vi "PSVCH_Engine.vi"() -> ()   [LabVIEW 2016]
uses:
  Ctrls/PSVCH_VCH Info.ctl
  Ctrls/PSVCH_Status.ctl
  ToolKit/Formula/Ctrls/PSFormula_FOR_Formula Node.ctl
  ToolKit/Formula/Ctrls/PSFormula_FOR_Formula Step.ctl
  ToolKit/Formula/Ctrls/PSFormula_FOR_Formula Para.ctl
  ToolKit/Formula/Ctrls/PSFormula_FOR_Formula MidVar Data.ctl
  Ctrls/PSVCH_VarList.ctl
  Ctrls/PSVCH_Formula Node.ctl
  Ctrls/PSVCH_Formula Step.ctl
  Ctrls/PSVCH_Formula Para.ctl
  Ctrls/PSVCH_Formula MidVar Data.ctl
  Ctrls/PSVCH_VCH Status.ctl
  Architecture/Queue Management/ARC_Queue Create_Single.vi
  Architecture/Queue Management/ARC_Queue Valid.vi
  Architecture/Queue Management/ARC_Queue Remove Element.vi
  Architecture/Queue Management/ARC_Queue Insert Element.vi
  Architecture/Queue Management/ARC_Queue Destroy_Single.vi
panel:
  in  "Formula Node":T1
  in  "Q-Caller":string
  in  "TempVariable":T12
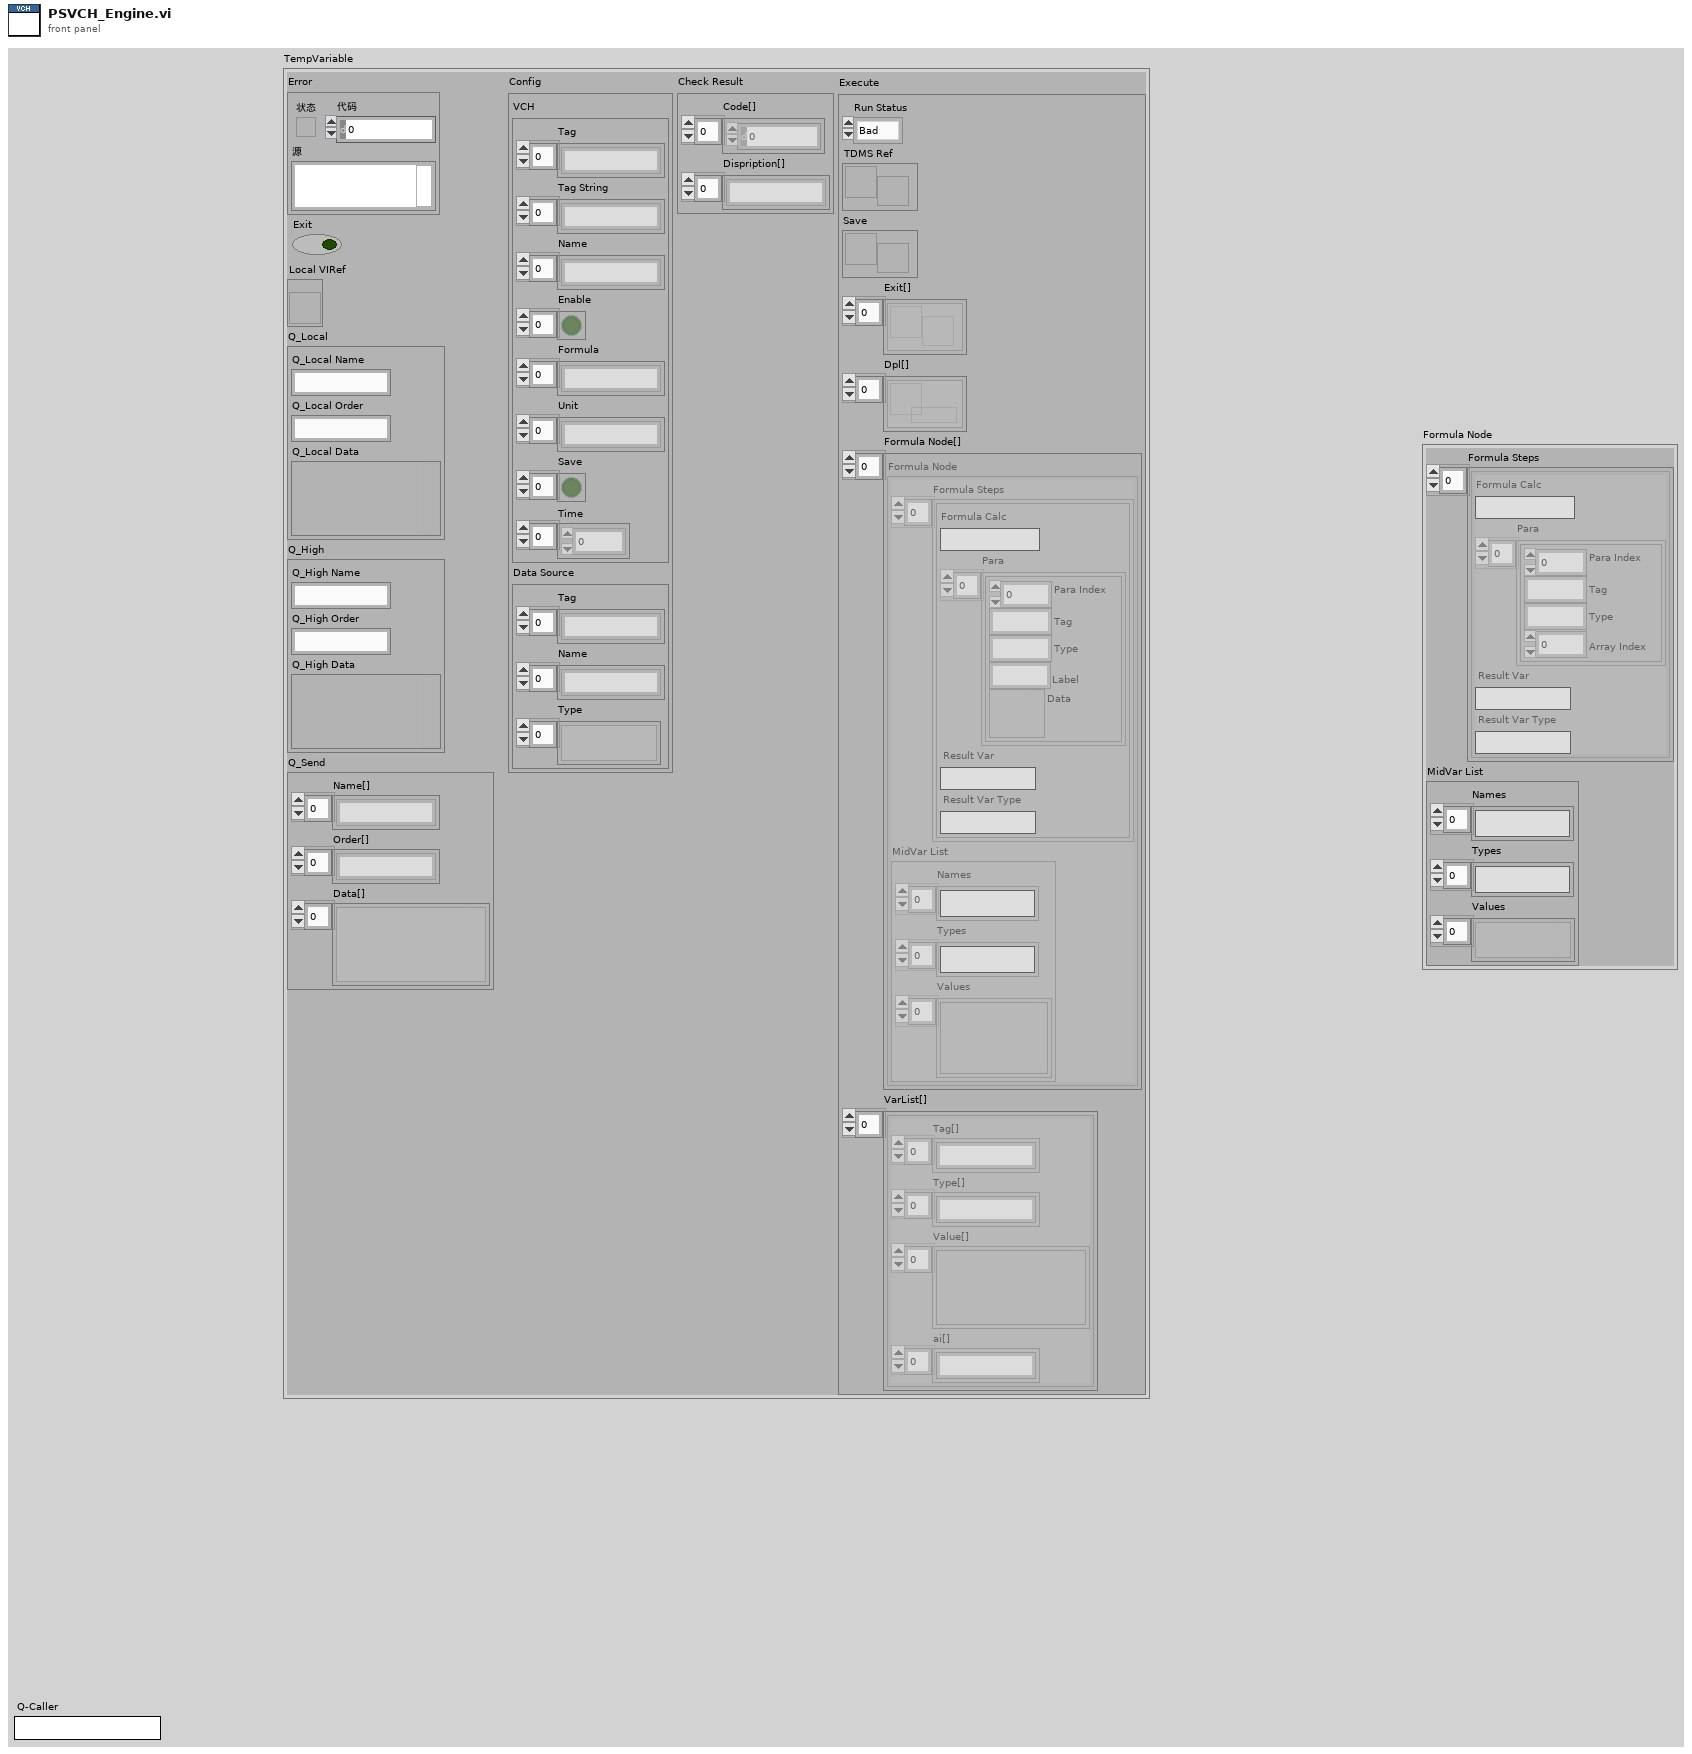
[diagram p1: front panel]
types:
  T1 = typedef "PSVCH_Formula Node.ctl" = cluster{"Formula Steps":T2[], "MidVar List":T4}
  T2 = typedef "PSVCH_Formula Step.ctl" = cluster{"Formula Calc":string, "Para":T3[], "Result Var":string, "Result Var Type":string}
  T3 = typedef "PSVCH_Formula Para.ctl" = cluster{"Para Index":i32, "Tag":string, "Type":string, "Array Index":i32}
  T4 = typedef "PSVCH_Formula MidVar Data.ctl" = cluster{"Names":string[], "Types":string[], "Values":variant[]}
  T5 = typedef "PSVCH_VCH Info.ctl" = cluster{"Tag":string[], "Tag String":string[], "Name":string[], "Enable":bool[], "Formula":string[], "Unit":string[], "Save":bool[], "Time":i64[]}
  T6 = typedef "PSVCH_Status.ctl" = enum16{"Bad", "Stop", "Run", "Pause"}
  T7 = typedef "PSFormula_FOR_Formula Node.ctl" = cluster{"Formula Steps":T8[], "MidVar List":T10}
  T8 = typedef "PSFormula_FOR_Formula Step.ctl" = cluster{"Formula Calc":string, "Para":T9[], "Result Var":string, "Result Var Type":string}
  T9 = typedef "PSFormula_FOR_Formula Para.ctl" = cluster{"Para Index":i32, "Tag":string, "Type":string, "Label":string, "Data":variant}
  T10 = typedef "PSFormula_FOR_Formula MidVar Data.ctl" = cluster{"Names":string[], "Types":string[], "Values":variant[]}
  T11 = typedef "PSVCH_VarList.ctl" = cluster{"Tag[]":string[], "Type[]":string[], "Value[]":variant[], "ai[]":string[]}
  T12 = cluster{"Error":errorcluster, "Exit":bool, "Local VIRef":refnum<vi>, "Q_Local":cluster{"Q_Local Name":string, "Q_Local Order":string, "Q_Local Data":variant}, "Q_High":cluster{"Q_High Name":string, "Q_High Order":string, "Q_High Data":variant}, "Q_Send":cluster{"Name[]":string[], "Order[]":string[], "Data[]":variant[]}, "Config":cluster{"VCH":T5, "Data Source":cluster{"Tag":string[], "Name":string[], "Type":variant[]}}, "Check Result":cluster{"Code[]":i32[], "Dispription[]":string[]}, "Execute":cluster{"Run Status":T6, "TDMS Ref":refnum<notifier>, "Save":refnum<notifier>, "Exit[]":refnum<notifier>[], "Dpl[]":refnum<queue>[], "Formula Node[]":T7[], "VarList[]":T11[]}}
  T13 = typedef "PSVCH_VCH Status.ctl" = cluster{"Tag":string[], "Code[]":i32[], "Dispription[]":string[]}
  T14 = cluster{"Q_High Name":string, "Tag":string, "t0":timestamp, "Period":i64, "Exit":refnum<notifier>, "Dpl":refnum<queue>, "TDMS Ref":refnum<notifier>, "Save":refnum<notifier>, "Formula Node 2":T7, "VarList":T11, "Save?":bool, "Name":string, "Unit":string}
  T15 = cluster{"Tag":string[], "Name":string[], "Type":variant[]}
  T16 = cluster{"Data Source":cluster{"Tag":string[], "Name":string[], "Type":variant[]}, "VCH":T5}
  T17 = cluster{"Q_Local Name":string, "Error":errorcluster}
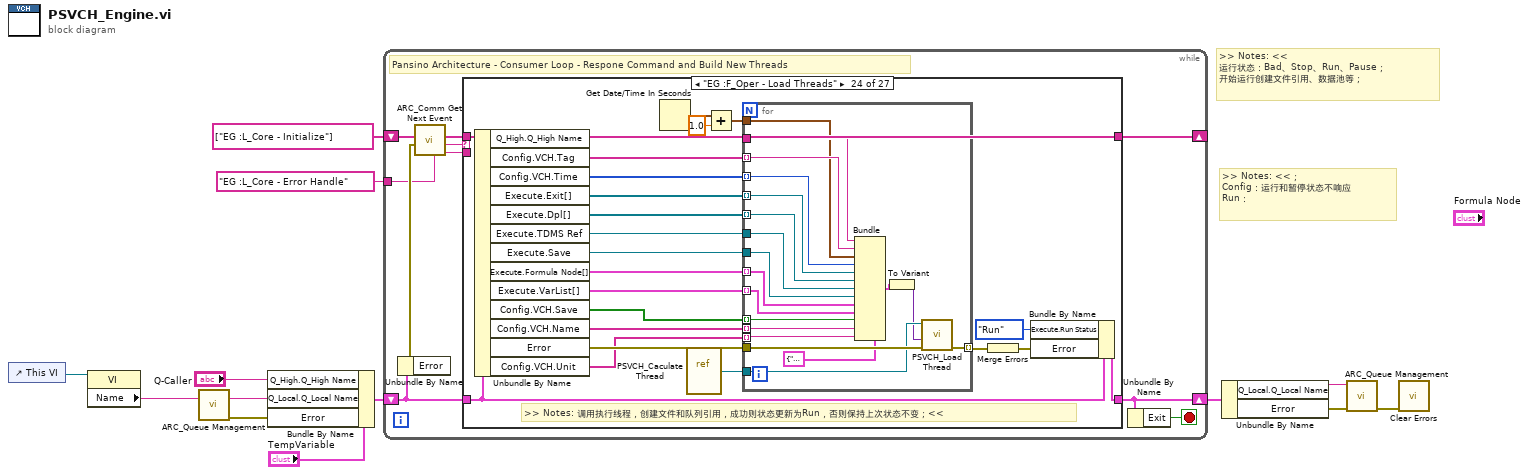
[diagram p0: block diagram]
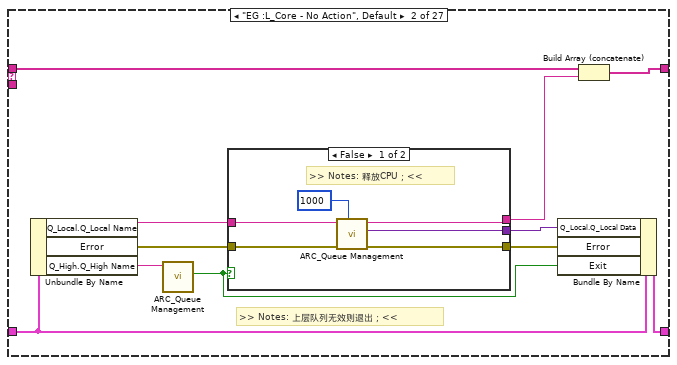
[diagram p3: hidden frame]
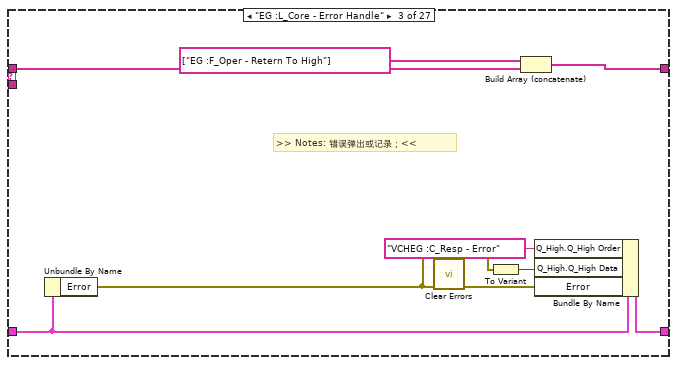
[diagram p5: hidden frame]
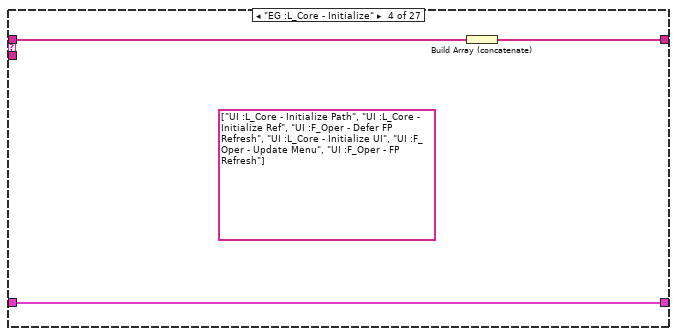
[diagram p6: hidden frame]
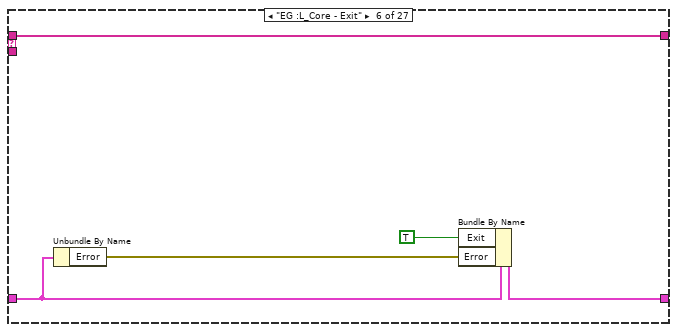
[diagram p8: hidden frame]
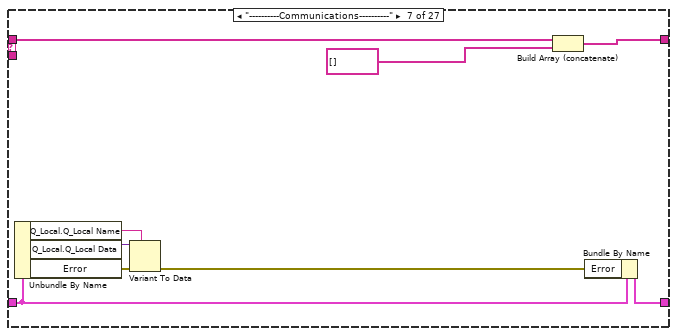
[diagram p9: hidden frame]
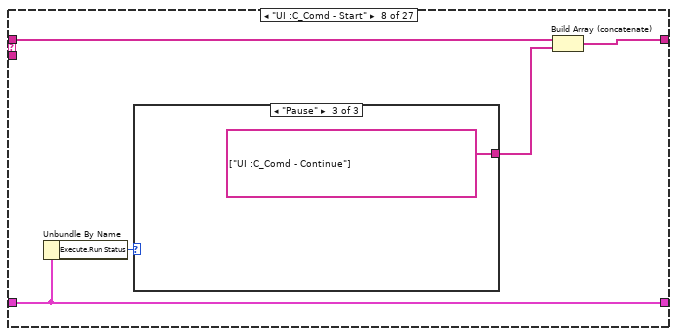
[diagram p10: hidden frame]
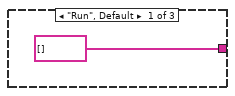
[diagram p11: hidden frame]
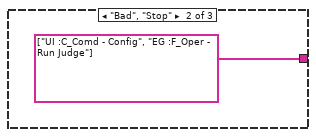
[diagram p12: hidden frame]
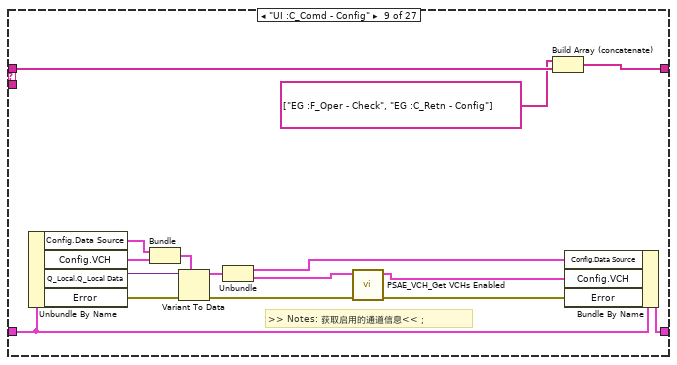
[diagram p13: hidden frame]
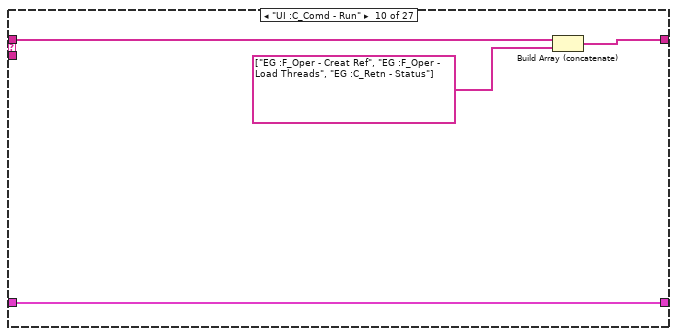
[diagram p14: hidden frame]
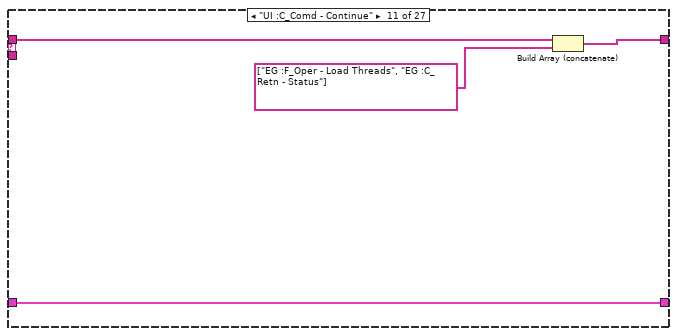
[diagram p15: hidden frame]
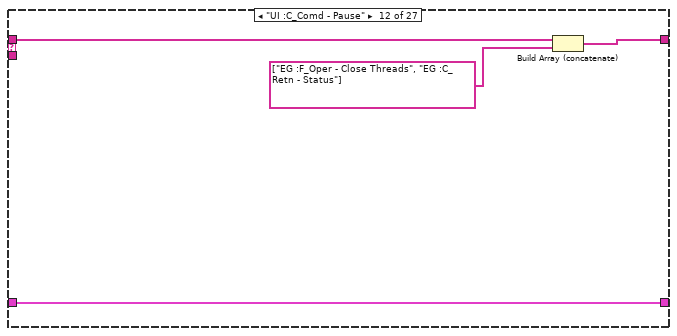
[diagram p16: hidden frame]
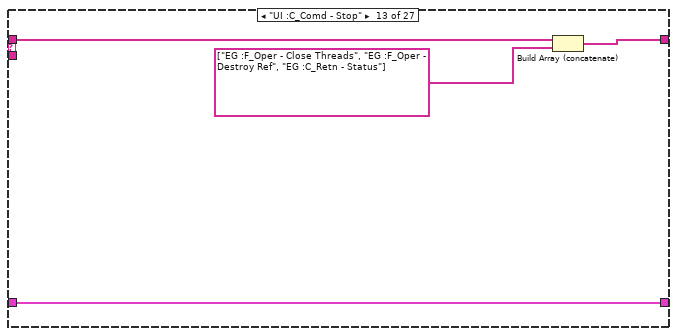
[diagram p17: hidden frame]
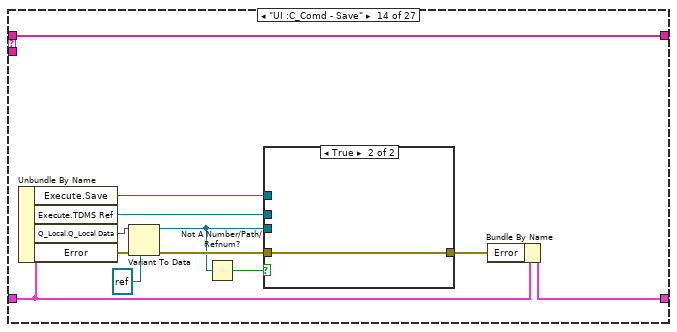
[diagram p18: hidden frame]
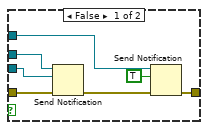
[diagram p19: hidden frame]
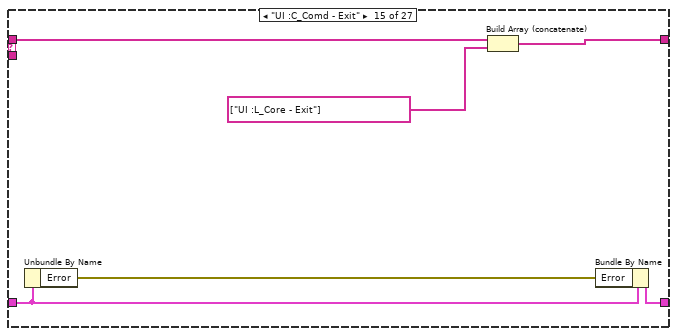
[diagram p20: hidden frame]
diagram:
  # ">> Notes: <<；\nConfig：运行和暂停状态不响应\nRun："
  # ">> Notes: <<\n运行状态：Bad、Stop、Run、Pause；\n开始运行创建文件引用、数据池等；"
  n1 = control-ref of="This VI"() -> (w2:refnum<vi>)
  n2 = property class="VI"(reference=w2) -> ("Name"=w1:string)  [unwired: 1 in, 2 out]
  n3 = call-poly "ARC_Queue Management.vi"("Queue Name"=w1) -> ("error out"=w3:errorcluster)  [unwired: 8 in, 2 out]
  n4 = Bundle By Name(cluster="TempVariable", "Q_High.Q_High Name"="Q-Caller", "Q_Local.Q_Local Name"=w1, "Error"=w3) -> (w11:T12)
  n5 = while {
    shift-right: [w16] -> w7
    shift-left: w11 -> [w18]
    shift-right: [w19] -> _
    shift-left: string[] ["EG :L_Core - Initialize"] -> [w22]
    tunnel: "EG :L_Core - Error Handle" ("Error Handle") -> [w14]
    stop <- w15 stop-if-true
    # "Pansino Architecture - Consumer Loop - Respone Command and Build New Threads"
    n6 = Unbundle By Name(w18) -> ("Error"=w17:errorcluster)
    n7 = call "ARC_Comm Get Next Event.vi"("Error Handle"=w14, "error in (no error)"=w17, "event queue in"=w22) -> ("prev event"=w13:string, "next event"=w21:string, "event queue out"=w20:string[])  [unwired: 3 in]
    n8 = case shown="\"EG :F_Oper - Load Threads\"" w21 {
      tunnel: w18 -> [w23 w32 w49 w53 w55 w58 w67 w72 w92 w95 w99 w103 w107 w121 w135 w148 w157 w171 w174 w183 w191 w225 w249 w279 w307 w327 w342]
      tunnel: w20 -> [w24 w30 w51 w54 w56 w61 w70 w75 w94 w98 w102 w106 w110 w122 w133 w149 w151 w160 w175 w184 w199 w223 w250 w282 w309 w328 w343]
      tunnel: [w24 w29 w45 w52 w56 w61 w69 w74 w93 w97 w101 w105 w109 w122 w132 w143 w150 w159 w175 w184 w199 w223 w250 w282 w309 w328 w337] -> w19
      tunnel: [w23 w31 w50 w53 w55 w59 w66 w72 w91 w95 w99 w103 w107 w119 w134 w147 w156 w170 w173 w182 w192 w224 w245 w280 w308 w323 w342] -> w16
      tunnel: w13 -> [_ _ _ _ _ _ _ _ _ _ _ _ _ _ _ _ _ _ _ _ _ _ _ _ _ _ _]
      frame "----------Core Status----------" {
      }
      frame "EG :L_Core - No Action", Default {
        # ">> Notes: 上层队列无效则退出；<<"
        n9 = Unbundle By Name(w32) -> ("Q_Local.Q_Local Name"=w27:string, "Error"=w33:errorcluster, "Q_High.Q_High Name"=w26:string)
        n10 = call-poly "ARC_Queue Management.vi"("Queue Name(unamed)"=w26) -> ("Not Exist?"=w25:bool)  [unwired: 8 in, 2 out]
        n11 = case shown="False" w25 {
          tunnel: [w41 w42] -> w35
          tunnel: [w40 _] -> w34
          tunnel: w33 -> [w39 w42]
          tunnel: [w38 _] -> w28
          tunnel: w27 -> [w37 _]
          frame False {
            # ">> Notes: 释放CPU；<<"
            n12 = call-poly "ARC_Queue Management.vi"("Time out(-1)_queue out"=1000, "error in (no error)"=w39, "Queue Name(unamed)"=w37) -> ("error out"=w41:errorcluster, "Data"=w40:variant, "Event"=w38:string)  [unwired: 5 in, 1 out]
          }
          frame True {
          }
        }
        n13 = Bundle By Name(cluster=w32, "Q_Local.Q_Local Data"=w34, "Error"=w35, "Exit"=w25) -> (w31:T12)
        n14 = Build Array (concatenate)(w30, w28) -> (w29:string[])
      }
      frame "EG :L_Core - Error Handle" {
        # ">> Notes: 错误弹出或记录；<<"
        n15 = Unbundle By Name(w49) -> ("Error"=w46:errorcluster)
        n16 = call <vilib>:"Clear Errors.vi"("error in (no error)"=w46) -> ("error out"=w47:errorcluster)  [unwired: 5 in, 1 out]
        n17 = To Variant(anything=w46) -> (Variant=w48:variant)
        n18 = Build Array (concatenate)(string[] ["EG :F_Oper - Retern To High"] ("数组"), w51) -> (w45:string[])
        n19 = Bundle By Name(cluster=w49, "Q_High.Q_High Order"="VCHEG :C_Resp - Error", "Q_High.Q_High Data"=w48, "Error"=w47) -> (w50:T12)
      }
      frame "EG :L_Core - Initialize" {
        (unwired) string[] ["UI :L_Core - Initialize Path", "UI :L_Core - Initialize Ref", "UI :F_Oper - Defer FP Refresh", "UI :L_Core - Initialize UI", "UI :F_Oper - Update Menu", "UI :F_Oper - FP Refresh"] ("数组")
        n20 = Build Array (concatenate)(w54) -> (w52:string[])
      }
      frame "EG :L_Core - Initialize Path" {
      }
      frame "EG :L_Core - Exit" {
        n21 = Unbundle By Name(w58) -> ("Error"=w60:errorcluster)
        n22 = Bundle By Name(cluster=w58, "Exit"=TRUE, "Error"=w60) -> (w59:T12)
      }
      frame "----------Communications----------" {
        n23 = Unbundle By Name(w67) -> ("Q_Local.Q_Local Name"=w62:string, "Q_Local.Q_Local Data"=w63:variant, "Error"=w65:errorcluster)
        n24 = Variant To Data(error in=w65, type=w62, Variant=w63) -> (error out=w64:errorcluster)  [unwired: 1 out]
        n25 = Build Array (concatenate)(w70, string[] [] ("数组")) -> (w69:string[])
        n26 = Bundle By Name(cluster=w67, "Error"=w64) -> (w66:T12)
      }
      frame "UI :C_Comd - Start" {
        n27 = Unbundle By Name(w72) -> ("Execute.Run Status"=w73:T6)
        n28 = case shown="\"Pause\"" w73 {
          tunnel: [string[] [] ("数组") string[] ["UI :C_Comd - Config", "EG :F_Oper - Run Judge"] ("数组") string[] ["UI :C_Comd - Continue"] ("数组")] -> w71
          frame "Run", Default {
          }
          frame "Bad", "Stop" {
          }
          frame "Pause" {
          }
        }
        n29 = Build Array (concatenate)(w75, w71) -> (w74:string[])
      }
      frame "UI :C_Comd - Config" {
        # ">> Notes: 获取启用的通道信息<<；"
        n30 = Unbundle By Name(w92) -> ("Config.Data Source"=w87:T15, "Config.VCH"=w88:T5, "Q_Local.Q_Local Data"=w89:variant, "Error"=w90:errorcluster)
        n31 = Bundle("Data Source"=w87, "VCH"=w88) -> (w86:T16)  [unwired: 1 in]
        n32 = Variant To Data(error in=w90, type=w86, Variant=w89) -> (data=w85:T16, error out=w83:errorcluster)
        n33 = Unbundle(w85) -> ("Data Source"=w84:T15, "VCH"=w82:T5)
        n34 = call "PSAE_VCH_Get VCHs Enabled.vi"("Error In"=w83, "VCH"=w82) -> ("Error Out"=w81:errorcluster, "VCH"=w80:T5)  [unwired: 8 in]
        n35 = Build Array (concatenate)(string[] ["EG :F_Oper - Check", "EG :C_Retn - Config"] ("数组"), w94) -> (w93:string[])
        n36 = Bundle By Name(cluster=w92, "Config.Data Source"=w84, "Config.VCH"=w80, "Error"=w81) -> (w91:T12)
      }
      frame "UI :C_Comd - Run" {
        n37 = Build Array (concatenate)(w98, string[] ["EG :F_Oper - Creat Ref", "EG :F_Oper - Load Threads", "EG :C_Retn - Status"] ("数组")) -> (w97:string[])
      }
      frame "UI :C_Comd - Continue" {
        n38 = Build Array (concatenate)(w102, string[] ["EG :F_Oper - Load Threads", "EG :C_Retn - Status"] ("数组")) -> (w101:string[])
      }
      frame "UI :C_Comd - Pause" {
        n39 = Build Array (concatenate)(w106, string[] ["EG :F_Oper - Close Threads", "EG :C_Retn - Status"] ("数组")) -> (w105:string[])
      }
      frame "UI :C_Comd - Stop" {
        n40 = Build Array (concatenate)(w110, string[] ["EG :F_Oper - Close Threads", "EG :F_Oper - Destroy Ref", "EG :C_Retn - Status"] ("数组")) -> (w109:string[])
      }
      frame "UI :C_Comd - Save" {
        n41 = Unbundle By Name(w121) -> ("Execute.Save"=w120:refnum<notifier>, "Execute.TDMS Ref"=w115:refnum<notifier>, "Q_Local.Q_Local Data"=w116:variant, "Error"=w117:errorcluster)
        n42 = Variant To Data(error in=w117, type=refnum<k34> refnum ("通知"), Variant=w116) -> (data=w112:refnum<k34>, error out=w113:errorcluster)
        n43 = Not A Number/Path/Refnum?(number/path/refnum=w112) -> (NaN/Path/Refnum?=w111:bool)
        n44 = case shown="True" w111 {
          tunnel: w120 -> [w129 _]
          tunnel: [w127 w130] -> w118
          tunnel: w115 -> [w126 _]
          tunnel: w113 -> [w125 w130]
          tunnel: w112 -> [w123 _]
          frame False {
            n45 = Send Notification(notification=w123, notifier=w126, error in (no error)=w125) -> (error out=w124:errorcluster)  [unwired: 1 out]
            n46 = Send Notification(notification=TRUE ("通知"), notifier=w129, error in (no error)=w124) -> (error out=w127:errorcluster)  [unwired: 1 out]
          }
          frame True {
          }
        }
        n47 = Bundle By Name(cluster=w121, "Error"=w118) -> (w119:T12)
      }
      frame "UI :C_Comd - Exit" {
        n48 = Unbundle By Name(w135) -> ("Error"=w136:errorcluster)
        n49 = Build Array (concatenate)(w133, string[] ["UI :L_Core - Exit"] ("数组")) -> (w132:string[])
        n50 = Bundle By Name(cluster=w135, "Error"=w136) -> (w134:T12)
      }
      frame "EG :C_Retn - Config" {
        n51 = Unbundle By Name(w148) -> ("Config.VCH.Tag"=w139:string[], "Check Result.Code[]"=w140:i32[], "Check Result.Dispription[]"=w141:string[], "Error"=w146:errorcluster)
        n52 = Bundle By Name(cluster=T13 {"Tag"=[], "Code[]"=[], "Dispription[]"=[]} ("输出簇"), "Tag"=w139, "Code[]"=w140, "Dispription[]"=w141) -> (w138:T13)
        n53 = To Variant(anything=w138) -> (Variant=w145:variant)
        n54 = Build Array (concatenate)(w149, "EG :F_Oper - Retern To High" ("Q_High.Q_High Order")) -> (w143:string[])
        n55 = Bundle By Name(cluster=w148, "Q_High.Q_High Order"="VCHEG :C_Resp - Config", "Q_High.Q_High Data"=w145, "Error"=w146) -> (w147:T12)
      }
      frame "EG :C_Retn - Status" {
        n56 = Unbundle By Name(w157) -> ("Execute.Run Status"=w154:T6)
        n57 = To Variant(anything=w154) -> (Variant=w155:variant)
        n58 = Bundle By Name(cluster=w157, "Q_High.Q_High Order"="VCHEG :C_Resp - Status", "Q_High.Q_High Data"=w155) -> (w156:T12)
        n59 = Build Array (concatenate)(w151, "EG :F_Oper - Retern To High" ("Q_High.Q_High Order")) -> (w150:string[])
      }
      frame "THx :C_Resp - Error" {
        # ">> Notes: 底层线程返回的错误及发生错误的线程的Tag/Q_Name，关闭引用；<<"
        n60 = Unbundle By Name(w171) -> ("Q_Local.Q_Local Name"=w168:string, "Error"=w165:errorcluster, "Q_Local.Q_Local Data"=w169:variant, "Error"=w167:errorcluster)
        n61 = Bundle("Q_Local Name"=w168, "Error"=w165) -> (w166:T17)  [unwired: 1 in]
        n62 = Variant To Data(error in=w167, type=w166, Variant=w169) -> (data=w164:T17, error out=w163:errorcluster)
        n63 = Unbundle(w164) -> ("Error"=w162:errorcluster)  [unwired: 1 out]
        n64 = Merge Errors(w162, w163) -> (w161:errorcluster)
        n65 = Build Array (concatenate)(w160, string[] ["EG :F_Oper - Close Threads", "EG :F_Oper - Destroy Ref", "EG :C_Retn - Status"] ("数组")) -> (w159:string[])
        n66 = Bundle By Name(cluster=w171, "Error"=w161) -> (w170:T12)
      }
      frame "----------Operations----------" {
        n67 = Unbundle By Name(w174) -> ("Error"=w172:errorcluster)
        n68 = Bundle By Name(cluster=w174, "Error"=w172) -> (w173:T12)
      }
      frame "EG :F_Oper - Retern To High" {
        n69 = Unbundle By Name(w183) -> ("Q_High.Q_High Name"=w177:string, "Q_High.Q_High Order"=w178:string, "Q_High.Q_High Data"=w179:variant, "Error"=w181:errorcluster)
        n70 = call-poly "ARC_Queue Management.vi"("Queue Name(unamed)"=w177) -> ("Not Exist?"=w176:bool)  [unwired: 8 in, 2 out]
        n71 = case shown="False" w176 {
          tunnel: w181 -> [w189 w190]
          tunnel: [w188 w190] -> w180
          tunnel: w179 -> [w187 _]
          tunnel: w178 -> [w186 _]
          tunnel: w177 -> [w185 _]
          frame False {
            n72 = call-poly "ARC_Queue Management.vi"("error in (no error)"=w189, "Data"=w187, "Event"=w186, "Queue Name(unamed)"=w185) -> ("error out"=w188:errorcluster)  [unwired: 6 in, 1 out]
          }
          frame True {
          }
        }
        n73 = Bundle By Name(cluster=w183, "Error"=w180) -> (w182:T12)
      }
      frame "EG :F_Oper - Send To Threads" {
        # ">> Notes: 发送指令给线程，可使用并行for循环提高同步性；<<"
        n74 = Unbundle By Name(w191) -> ("Q_Send.Name[]"=w193:string[], "Q_Send.Order[]"=w195:string[], "Q_Send.Data[]"=w196:variant[], "Error"=w194:errorcluster)
        n75 = for {
          tunnel: w193 -> [w205] mode=indexing
          tunnel: w194 -> [w208]
          tunnel: w195 -> [w207]
          tunnel: w196 -> [w206]
          tunnel: [w202] -> w197 mode=indexing
          i -> [w201]
          n76 = Index Array(array=w207, index=w201) -> (element=w204:string)
          n77 = Index Array(array=w206, index=w201) -> (element=w203:variant)
          n78 = call-poly "ARC_Queue Management.vi"("Time out(-1)_queue in"=50, "error in (no error)"=w208, "Data"=w203, "Event"=w204, "Queue Name(unamed)"=w205) -> ("error out"=w202:errorcluster)  [unwired: 5 in, 1 out]
        }
        n79 = Merge Errors(w197) -> (w198:errorcluster)
        n80 = Bundle By Name(cluster=w191, "Error"=w198) -> (w192:T12)
      }
      frame "EG :F_Oper - Check" {
        # ">> Notes: 执行公式检查,生成公式节点、更新状态；<<"
        n81 = Unbundle By Name(w225) -> ("Config.VCH.Formula"=w215:string[], "Config.Data Source"=w221:T15, "Error"=w216:errorcluster)
        n82 = for {
          tunnel: w216 -> [w232]
          tunnel: [w231] -> w222 mode=indexing
          tunnel: w221 -> [_]
          tunnel: w215 -> [w230] mode=indexing
          tunnel: [w227] -> w214 mode=indexing
          tunnel: [w229] -> w218 mode=indexing
          tunnel: [w228] -> w219 mode=indexing
          tunnel: [w226] -> w217 mode=indexing
          n83 = call "PSVCH_Formula Check.vi"("Error In"=w232, "Formula"=w230) -> ("Error Out"=w231:errorcluster, "Formula Node out"=w228:T7, "source"=w229:string, "code"=w227:i32, "VarList"=w226:T11)  [unwired: 5 in]
        }
        n84 = Equal To 0?(x=w214) -> (x = 0?=w213:bool[])
        n85 = And Array Elements(Boolean array=w213) -> (logical AND=w212:bool)
        n86 = Select(t=PSVCH_Status."Stop" ("Execute.Run Status"), s=w212, f=PSVCH_Status."Bad") -> (s? t:f=w210:T6)
        n87 = Merge Errors(w222) -> (w220:errorcluster)
        n88 = Bundle By Name(cluster=w225, "Execute.Run Status"=w210, "Execute.VarList[]"=w217, "Check Result.Code[]"=w214, "Check Result.Dispription[]"=w218, "Execute.Formula Node[]"=w219, "Error"=w220) -> (w224:T12)
      }
      frame "EG :F_Oper - Creat Ref" {
        w238 = FALSE ("Exit")
        # ">> Notes: 创建数据池引用、文件引用等，更新状态<<"
        n89 = Unbundle By Name(w249) -> ("Config.VCH.Tag"=w247:string[], "Error"=w248:errorcluster)
        n90 = for {
          tunnel: w248 -> [w259]
          tunnel: w247 -> [w257] mode=indexing
          tunnel: waveform(dbl)[] [] ("Out") -> [w258]
          tunnel: [w256] -> w243 mode=indexing
          tunnel: [w255] -> w246 mode=indexing
          tunnel: [w254] -> w242 mode=indexing
          n91 = Obtain Queue(max queue size (-1, unlimited)=1 ("队列最大值（-1，无限）"), name (unnamed)=w257, element data type=w258, error in (no error)=w259) -> (queue out=w256:refnum<queue>, error out=w252:errorcluster)  [unwired: 1 in, 1 out]
          n92 = Obtain Notifier(name (unnamed)=w257, notification data type=FALSE ("Exit"), error in (no error)=w252) -> (notifier out=w254:refnum<notifier>, error out=w255:errorcluster)  [unwired: 1 in, 1 out]
        }
        n93 = Merge Errors(w246) -> (w241:errorcluster)
        n94 = Obtain Notifier(notification data type=w238, error in (no error)=w241) -> (notifier out=w240:refnum<notifier>, error out=w239:errorcluster)  [unwired: 2 in, 1 out]
        n95 = Send Notification(notification=w238, notifier=w240, error in (no error)=w239) -> (notifier out=w237:refnum<notifier>, error out=w236:errorcluster)
        n96 = Obtain Notifier(notification data type=refnum<k34> refnum ("通知"), error in (no error)=w236) -> (notifier out=w233:refnum<notifier>, error out=w235:errorcluster)  [unwired: 2 in, 1 out]
        n97 = Bundle By Name(cluster=w249, "Execute.Dpl[]"=w243, "Execute.Exit[]"=w242, "Execute.Save"=w237, "Execute.TDMS Ref"=w233, "Error"=w235) -> (w245:T12)
      }
      frame "EG :F_Oper - Load Threads" {
        # ">> Notes: 调用执行线程，创建文件和队列引用，成功则状态更新为Run，否则保持上次状态不变；<<"
        n98 = Unbundle By Name(w279) -> ("Q_High.Q_High Name"=w275:string, "Config.VCH.Tag"=w274:string[], "Config.VCH.Time"=w265:i64[], "Execute.Exit[]"=w269:refnum<notifier>[], "Execute.Dpl[]"=w268:refnum<queue>[], "Execute.TDMS Ref"=w264:refnum<notifier>, "Execute.Save"=w263:refnum<notifier>, "Execute.Formula Node[]"=w267:T7[], "Execute.VarList[]"=w266:T11[], "Config.VCH.Save"=w262:bool[], "Config.VCH.Name"=w261:string[], "Error"=w281:errorcluster, "Config.VCH.Unit"=w260:string[])
        n99 = Get Date/Time In Seconds() -> (seconds since 1Jan1904=w273:timestamp)
        n100 = vi-ref "PSVCH_Caculate Thread.vi"() -> (w278:refnum<vi>)
        n101 = Add(x=w273, y=1.0) -> (x+y=w271:timestamp)
        n102 = for {
          tunnel: w281 -> [w301]
          tunnel: [w299] -> w277 mode=indexing
          tunnel: w278 -> [w300]
          tunnel: w274 -> [w297] mode=indexing
          tunnel: w275 -> [w298]
          tunnel: w271 -> [w292]
          tunnel: w269 -> [w294] mode=indexing
          tunnel: w268 -> [w293] mode=indexing
          tunnel: w267 -> [w288] mode=indexing
          tunnel: w266 -> [w289] mode=indexing
          tunnel: w265 -> [w291] mode=indexing
          tunnel: w264 -> [w290]
          tunnel: w263 -> [w287]
          tunnel: w262 -> [w286] mode=indexing
          tunnel: w261 -> [w285] mode=indexing
          tunnel: w260 -> [w283] mode=indexing
          n103 = Bundle(cluster=T14 {"Q_High Name"="", "Tag"="", "t0"=timestamp(0 s since 1904-01-01), "Period"=0, "Exit"=refnum, "Dpl"=refnum, "TDMS Ref"=refnum, "Save"=refnum, "Formula Node 2"={"Formula Steps"=[], "MidVar List"={"Names"=[], "Types"=[], "Values"=[]}}, "VarList"={"Tag[]"=[], "Type[]"=[], "Value[]"=[], "ai[]"=[]}, "Save?"=FALSE, "Name"="", "Unit"=""} ("Para"), "Q_High Name"=w298, "Tag"=w297, "t0"=w292, "Period"=w291, "Exit"=w294, "Dpl"=w293, "TDMS Ref"=w290, "Save"=w287, "Formula Node 2"=w288, "VarList"=w289, "Save?"=w286, "Name"=w285, "Unit"=w283) -> (w296:T14)
          n104 = To Variant(anything=w296) -> (Variant=w295:variant)
          n105 = call "PSVCH_Load Thread.vi"("Error In"=w301, "Control Value"=w295, "VIRef"=w300) -> ("Error Out"=w299:errorcluster)  [unwired: 7 in, 1 out]
        }
        n106 = Merge Errors(w277) -> (w276:errorcluster)
        n107 = Bundle By Name(cluster=w279, "Execute.Run Status"=PSVCH_Status."Run" ("Core.Run Status"), "Error"=w276) -> (w280:T12)
      }
      frame "EG :F_Oper - Close Threads" {
        # ">> Notes: 发送退出通知、关闭执行线程；<<"
        n108 = Unbundle By Name(w307) -> ("Execute.Exit[]"=w304:refnum<notifier>[], "Error"=w306:errorcluster)
        n109 = for {
          tunnel: w306 -> [w313]
          tunnel: [w312] -> w305 mode=indexing
          tunnel: w304 -> [w311] mode=indexing
          n110 = Send Notification(notification=TRUE ("强制销毁？(F)"), notifier=w311, error in (no error)=w313) -> (error out=w312:errorcluster)  [unwired: 1 out]
        }
        n111 = Merge Errors(w305) -> (w303:errorcluster)
        n112 = Bundle By Name(cluster=w307, "Execute.Run Status"=PSVCH_Status."Pause", "Error"=w303) -> (w308:T12)
      }
      frame "EG :F_Oper - Destroy Ref" {
        w314 = TRUE ("强制销毁？(F)")
        # ">> Notes: 清除引用无效时报错<<"
        # ">> Notes: 销毁数据池、文件等引用，更新状态<<"
        n113 = Unbundle By Name(w327) -> ("Execute.TDMS Ref"=w317:refnum<notifier>, "Execute.Save"=w319:refnum<notifier>, "Execute.Exit[]"=w321:refnum<notifier>[], "Execute.Dpl[]"=w325:refnum<queue>[], "Error"=w326:errorcluster)
        n114 = for {
          tunnel: w326 -> [w334]
          tunnel: w325 -> [w333] mode=indexing
          tunnel: [w331] -> w324 mode=indexing
          tunnel: w321 -> [w330] mode=indexing
          w329 = TRUE ("强制销毁？(F)")
          n115 = Release Queue(queue=w333, force destroy? (F)=w329, error in (no error)=w334) -> (error out=w332:errorcluster)  [unwired: 2 out]
          n116 = Release Notifier(notifier=w330, force destroy? (F)=w329, error in (no error)=w332) -> (error out=w331:errorcluster)  [unwired: 2 out]
        }
        n117 = Merge Errors(w324) -> (w320:errorcluster)
        n118 = Release Notifier(notifier=w319, force destroy? (F)=w314, error in (no error)=w320) -> (error out=w316:errorcluster)  [unwired: 2 out]
        n119 = Release Notifier(notifier=w317, force destroy? (F)=w314, error in (no error)=w316) -> (error out=w315:errorcluster)  [unwired: 2 out]
        n120 = call <vilib>:"Clear Errors.vi"("error in (no error)"=w315) -> ("error out"=w318:errorcluster)  [unwired: 5 in, 1 out]
        n121 = Bundle By Name(cluster=w327, "Error"=w318, "Execute.Run Status"=PSVCH_Status."Stop" ("Core.Run Status")) -> (w323:T12)
      }
      frame "EG :F_Oper - Run Judge" {
        n122 = Unbundle By Name(w342) -> ("Execute.Run Status"=w341:T6)
        n123 = Equal?(x=w341, y=PSVCH_Status."Stop") -> (x = y?=w339:bool)
        n124 = Select(t=string[] ["EG :F_Oper - Creat Ref", "EG :F_Oper - Load Threads", "EG :C_Retn - Status"] ("数组"), s=w339, f=string[] []) -> (s? t:f=w336:string[])
        n125 = Build Array (concatenate)(w343, w336) -> (w337:string[])
      }
    }
    n126 = Unbundle By Name(w16) -> ("Exit"=w15:bool)
  }
  n127 = Unbundle By Name(w7) -> ("Q_Local.Q_Local Name"=w10:string, "Error"=w8:errorcluster)
  n128 = call-poly "ARC_Queue Management.vi"("error in (no error)"=w8, "Queue Name(unamed)"=w10) -> ("error out"=w5:errorcluster)  [unwired: 7 in, 2 out]
  n129 = call <vilib>:"Clear Errors.vi"("error in (no error)"=w5) -> ()  [unwired: 5 in, 2 out]
